vi "Release-UI-references.vi"(8 "error in (no error)":errorcluster, 11 "Object ref in":T1) -> (0 "error out":errorcluster, 3 "Object ref out":T1)   [LabVIEW 2013, in "PowderDeposition.lvlib" / "PD-Main.lvclass"]
uses:
  PD-Main.lvclass
  Object-reference.ctl
  PD-Main.lvclass/PD-Main.ctl
  Read Actions.vi
  Read Motors-selection.vi
  Read Motors-status.vi
  Read Options.vi
  Read Motor sequences.vi
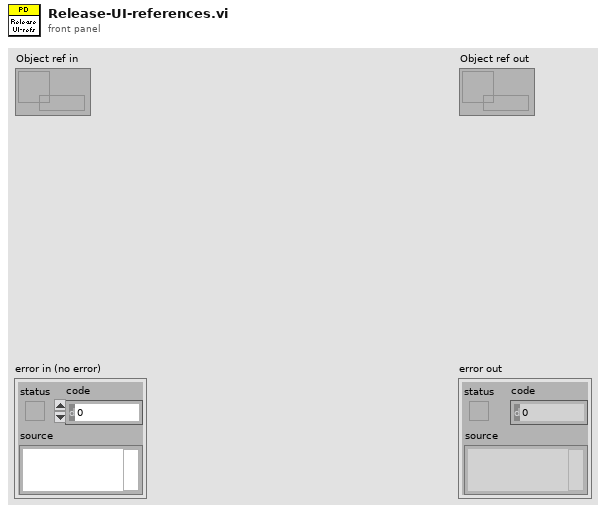
[diagram p1: front panel]
types:
  T1 = typedef "PowderDeposition.lvlib/PD-Main.lvclass/Object-reference.ctl" = refnum<data-value>
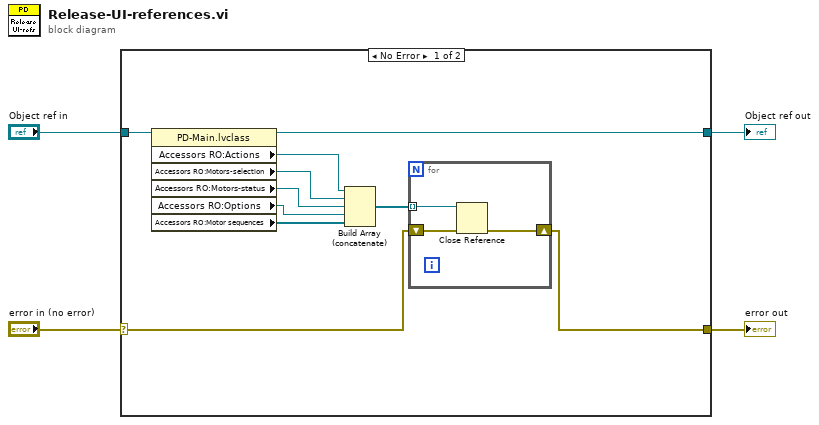
[diagram p0: block diagram]
diagram:
  n1 = case shown="No Error" "error in (no error)" {
    selector: "error in (no error)" -> [w6 w19]
    tunnel: [w5 w19] -> w3
    tunnel: [w13 w18] -> w1
    tunnel: "Object ref in" -> [w14 w18]
    frame No Error {
      n2 = property class="PD-Main.lvclass"(reference=w14) -> (reference out=w13:T1, "Accessors RO:Actions"=w12:refnum<vi>, "Accessors RO:Motors-selection"=w11:refnum<vi>, "Accessors RO:Motors-status"=w10:refnum<vi>, "Accessors RO:Options"=w9:refnum<vi>, "Accessors RO:Motor sequences"=w8:refnum<vi>[])  [unwired: 1 in, 1 out]
      n3 = Build Array (concatenate)(w12, w11, w10, w9, w8) -> (w7:refnum<vi>[])
      n4 = for {
        tunnel: w7 -> [w17] mode=indexing
        shift-right: [w15] -> w5
        shift-left: w6 -> [w16]
        n5 = Close Reference(reference=w17, error in (no error)=w16) -> (error out=w15:errorcluster)
      }
    }
    frame Error {
    }
  }
  "error out" <- w3
  "Object ref out" <- w1
